vi "Create Sample Timing.vi"(5 "Last OFDM symbol index":u16, 9 "packet start":bool, 10 "input valid":bool, 11 "channels in":T1) -> (0 "Cluster":T2, 1 "last sample":bool, 3 "channels out":T1)   [LabVIEW 2020]
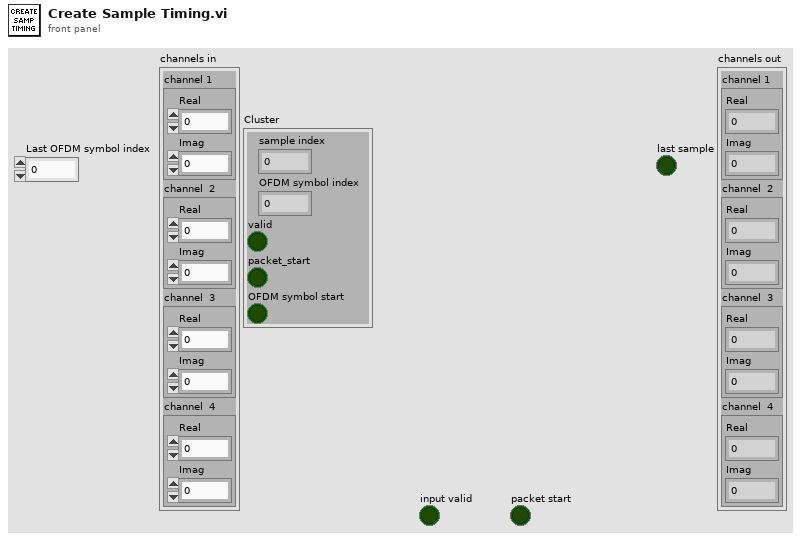
[diagram p1: front panel]
types:
  T1 = cluster{"channel 1 ":cluster{"Real":fxp<+/-,16,3>, "Imag":fxp<+/-,16,3>}, "channel  2":cluster{"Real":fxp<+/-,16,3>, "Imag":fxp<+/-,16,3>}, "channel  3":cluster{"Real":fxp<+/-,16,3>, "Imag":fxp<+/-,16,3>}, "channel  4":cluster{"Real":fxp<+/-,16,3>, "Imag":fxp<+/-,16,3>}}
  T2 = cluster{"sample index":u16, "OFDM symbol index":u16, "valid":bool, "packet_start":bool, "OFDM symbol start":bool}
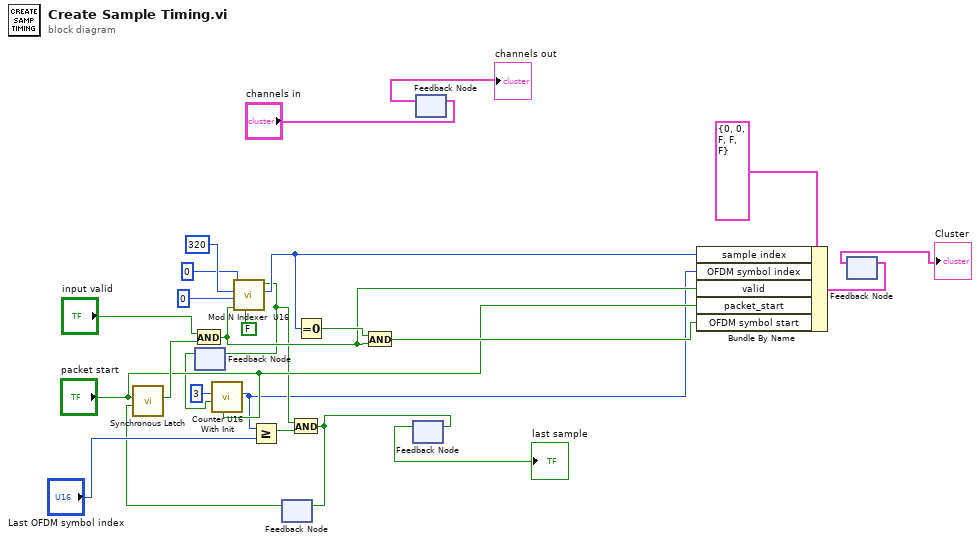
[diagram p0: block diagram]
diagram:
  n1 = feedback #1() -> (w4:bool)  [unwired: 1 in]
  n2 = call "Counter U16 With Init.vi"("reset"="packet start", "increment"=w4, "inintial value"=u16 3) -> ("count"=w2:u16)  [unwired: 8 in]
  n3 = Greater Or Equal?(x=w2, y="Last OFDM symbol index") -> (x >= y?=w18:bool)
  n4 = feedback #2() -> (w17:bool)  [unwired: 1 in]
  n5 = call "Synchronous Latch.vi"("clear"=w17, "set"="packet start") -> ("out"=w20:bool)  [unwired: 9 in]
  n6 = And(x="input valid", y=w20) -> (x .and. y?=w7:bool)
  n7 = call "Mod N Indexer  U16.vi"("reset"=FALSE, "enable"=w7, "reset value"=u16 0, "N"=u16 320, "initial value"=u16 0) -> ("index"=w10:u16, "wrap back"=w3:bool)  [unwired: 3 in, 2 out]
  n8 = feedback-in #1(w3) -> ()
  n9 = And(x=w3, y=w18) -> (x .and. y?=w16:bool)
  n10 = feedback-in #2(w16) -> ()
  n11 = Equal To 0?(x=w10) -> (x = 0?=w9:bool)
  n12 = And(x=w9, y=w7) -> (x .and. y?=w8:bool)
  n13 = feedback #3() -> (→"last sample":bool)  [unwired: 1 in]
  n14 = feedback-in #3(w16) -> ()
  n15 = feedback #4() -> (→"channels out":T1)  [unwired: 1 in]
  n16 = feedback-in #4("channels in") -> ()
  n17 = Bundle By Name(cluster=T2 {"sample index"=0, "OFDM symbol index"=0, "valid"=FALSE, "packet_start"=FALSE, "OFDM symbol start"=FALSE}, "sample index"=w10, "OFDM symbol index"=w2, "valid"=w7, "packet_start"="packet start", "OFDM symbol start"=w8) -> (w23:T2)
  n18 = feedback #5() -> (→"Cluster":T2)  [unwired: 1 in]
  n19 = feedback-in #5(w23) -> ()
